vi "coerce_to_ramp.vi"(1 "Requested speed\n(native units)":dbl format="%#_13g", 2 "Max Acceleration\n(native units)/second":dbl=72000.0 format="%#_13g") -> (0 "Ramped speed\n(percent)":dbl format="%#_13g")   [LabVIEW 2017]
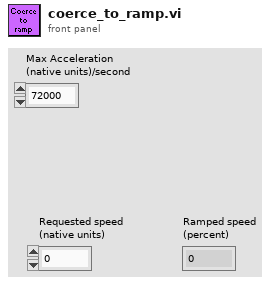
[diagram p1: front panel]
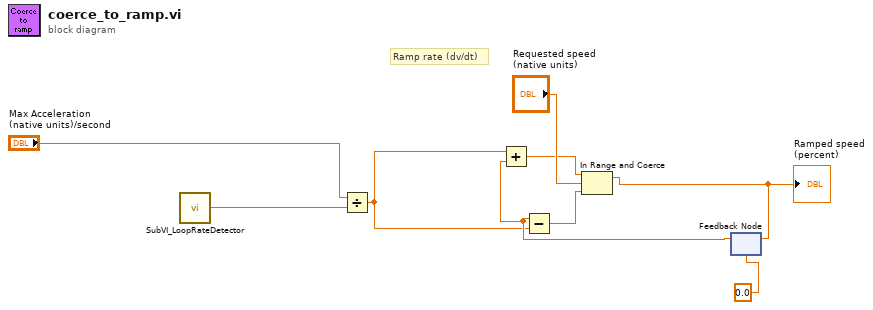
[diagram p0: block diagram]
diagram:
  # "Ramp rate (dv/dt)"
  n1 = call "SubVI_LoopRateDetector.vi"() -> ("loop rate (ms)"=w3:dbl)
  n2 = Divide(x="Max Acceleration\n(native units)/second", y=w3) -> (x/y=w1:dbl)
  n3 = feedback #1(0.0) -> (w6:dbl)
  n4 = Add(x=w1, y=w6) -> (x+y=w5:dbl)
  n5 = Subtract(x=w6, y=w1) -> (x-y=w7:dbl)
  n6 = In Range and Coerce(upper limit=w5, x="Requested speed\n(native units)", lower limit=w7) -> (coerced(x)=w4:dbl)  [unwired: 1 out]
  "Ramped speed\n(percent)" <- w4
  n7 = feedback-in #1(w4) -> ()
